vi "Get kb From Two Points.vi"(8 "error in (no error)":errorcluster caption="错误输入（无错误）", 10 "EndPointB":refnum<class "Point.lvclass">, 11 "EndPointA":refnum<class "Point.lvclass">) -> (0 "error out":errorcluster caption="错误输出", 1 "PerToXAxis":bool, 2 "b":dbl, 3 "k":dbl)   [LabVIEW 2011, in "Line.lvclass"]
uses:
  Line.lvclass
  Point/Point.lvclass
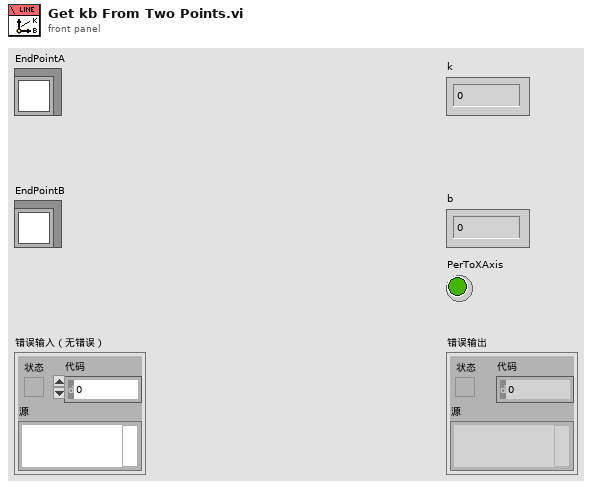
[diagram p1: front panel]
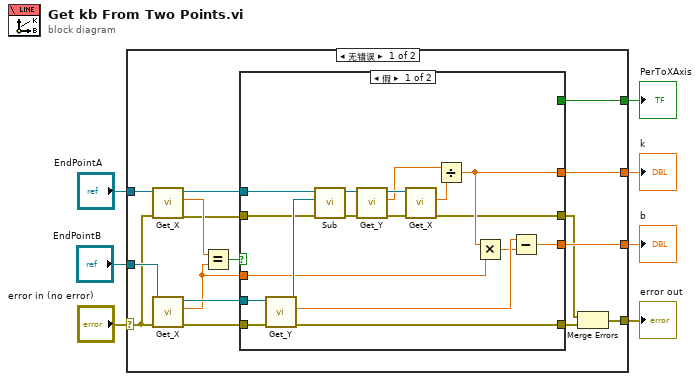
[diagram p0: block diagram]
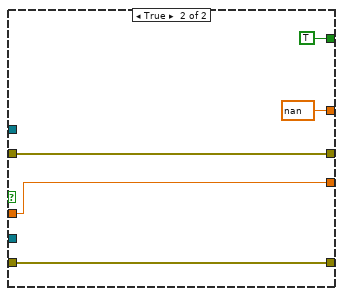
[diagram p2: hidden frame]
diagram:
  n1 = case shown="无错误" "error in (no error)" {
    selector: "error in (no error)" -> [w13 w47]
    tunnel: [w8 w47] -> w6
    tunnel: "EndPointA" -> [w23 _]
    tunnel: "EndPointB" -> [w22 _]
    tunnel: [w20 _] -> w3
    tunnel: [w18 _] -> w2
    tunnel: [w17 _] -> w1
    frame No Error {
      n2 = call "Get_X.vi"("error in (no error)"=w13, "Point输入"=w23) -> ("error out"=w11:errorcluster, "X"=w19:dbl, "Point输出"=w16:refnum<class "Point.lvclass">)  [unwired: 7 in]
      n3 = call "Get_X.vi"("error in (no error)"=w13, "Point输入"=w22) -> ("error out"=w12:errorcluster, "X"=w14:dbl, "Point输出"=w15:refnum<class "Point.lvclass">)  [unwired: 7 in]
      n4 = Equal?(x=w19, y=w14) -> (x = y?=w21:bool)
      n5 = case shown="假" w21 {
        tunnel: [w32 nan ("k")] -> w20
        tunnel: [w28 w42] -> w18
        tunnel: [_ TRUE ("PerToXAxis")] -> w17
        tunnel: w16 -> [w41 _]
        tunnel: w15 -> [w34 _]
        tunnel: w14 -> [w31 w42]
        tunnel: w12 -> [w27 w44]
        tunnel: w11 -> [w26 w43]
        tunnel: [w25 w43] -> w10
        tunnel: [w24 w44] -> w9
        frame False {
          n6 = call "Get_Y.vi"("error in (no error)"=w27, "Point输入"=w34) -> ("error out"=w24:errorcluster, "Y"=w30:dbl, "Point输出"=w33:refnum<class "Point.lvclass">)  [unwired: 7 in]
          n7 = call "Sub.vi"("error in (no error)"=w26, 10:"Point 输入"=w33, 11:"Point 输入"=w41) -> ("error out"=w39:errorcluster, "Point 输出"=w40:refnum<class "Point.lvclass">)  [unwired: 7 in]
          n8 = call "Get_Y.vi"("error in (no error)"=w39, "Point输入"=w40) -> ("error out"=w37:errorcluster, "Y"=w36:dbl, "Point输出"=w38:refnum<class "Point.lvclass">)  [unwired: 7 in]
          n9 = call "Get_X.vi"("error in (no error)"=w37, "Point输入"=w38) -> ("error out"=w25:errorcluster, "X"=w35:dbl)  [unwired: 7 in, 1 out]
          n10 = Divide(x=w36, y=w35) -> (x/y=w32:dbl)
          n11 = Multiply(x=w32, y=w31) -> (x*y=w29:dbl)
          n12 = Subtract(x=w30, y=w29) -> (x-y=w28:dbl)
        }
        frame True {
        }
      }
      n13 = Merge Errors(w10, w9) -> (w8:errorcluster)
    }
    frame Error {
    }
  }
  "error out" <- w6
  "k" <- w3
  "b" <- w2
  "PerToXAxis" <- w1
